vi "sv_Get NI Property Name String.vi"(7 "property":T1 items=["Channel name", "Channel description", "Axis label", "Unit string", "Waveform X-axis label", "Waveform X-axis unit string", "x0", "dx", "Number of samples", "X channel", "Filter settled", "dB reference", "Window", "Window parameter", "Window size", "FFT size", "Peak units", "Spectrum type", "Magnitude scale", "Spectral density", "Sensor sensitivity (mV/EU)", "X-axis dimension", "LabVIEW datatype", "Function type", "Function subtype", "X values", "Independent channel", "Column index", "Collection name", "Collection ID", "X Columns", "Phase unwrapped", "Sensor type", "Sensor maximum", "Averaging mode"]) -> (6 "TDMS property name":string, 10 "WDT attribute name":string)   [LabVIEW 2017]
uses:
  <vilib>/addons/_NISVFA/_Shared subVIs/Controls/NI Channel Properties.ctl
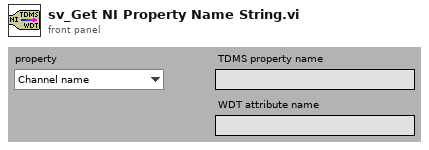
[diagram p1: front panel]
types:
  T1 = typedef "NI Channel Properties.ctl" = u16
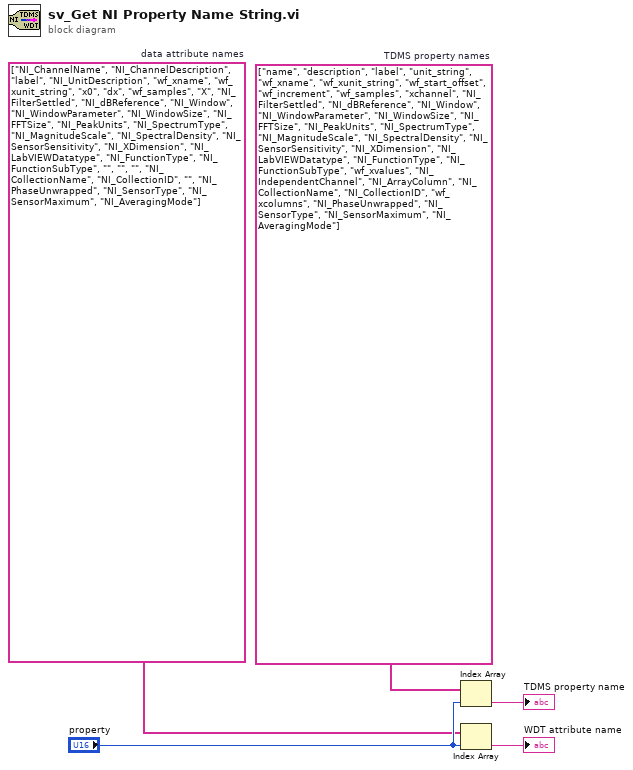
[diagram p0: block diagram]
diagram:
  w4 = string[] ["NI_ChannelName", "NI_ChannelDescription", "label", "NI_UnitDescription", "wf_xname", "wf_xunit_string", "x0", "dx", "wf_samples", "X", "NI_FilterSettled", "NI_dBReference", "NI_Window", "NI_WindowParameter", "NI_WindowSize", "NI_FFTSize", "NI_PeakUnits", "NI_SpectrumType", "NI_MagnitudeScale", "NI_SpectralDensity", "NI_SensorSensitivity", "NI_XDimension", "NI_LabVIEWDatatype", "NI_FunctionType", "NI_FunctionSubType", "", "", "", "NI_CollectionName", "NI_CollectionID", "", "NI_PhaseUnwrapped", "NI_SensorType", "NI_SensorMaximum", "NI_AveragingMode"]  # data attribute names
  w3 = string[] ["name", "description", "label", "unit_string", "wf_xname", "wf_xunit_string", "wf_start_offset", "wf_increment", "wf_samples", "xchannel", "NI_FilterSettled", "NI_dBReference", "NI_Window", "NI_WindowParameter", "NI_WindowSize", "NI_FFTSize", "NI_PeakUnits", "NI_SpectrumType", "NI_MagnitudeScale", "NI_SpectralDensity", "NI_SensorSensitivity", "NI_XDimension", "NI_LabVIEWDatatype", "NI_FunctionType", "NI_FunctionSubType", "wf_xvalues", "NI_IndependentChannel", "NI_ArrayColumn", "NI_CollectionName", "NI_CollectionID", "wf_xcolumns", "NI_PhaseUnwrapped", "NI_SensorType", "NI_SensorMaximum", "NI_AveragingMode"]  # TDMS property names
  n1 = Index Array(array=w3, index="property") -> (element=→"TDMS property name":string)
  n2 = Index Array(array=w4, index="property") -> (element=→"WDT attribute name":string)
